vi "CODMn线性公式.vi"(0 "标液浓度":dbl[](array[numeric]), 1 "信号值":dbl[](array[numeric]), 4 "启用":bool[](array[boolean]), 5 "method":T1 caption="方法" items=["最小二乘", "最小绝对残差", "Bisquare"], 6 "模型":enum32{"线性", "多项式", "折线"}(ring), 7 "精度":i32=6) -> (13 "Polynomial Coefficients 2":dbl[](array[numeric]) caption="多项式系数2", 14 "拟合方程":string, 15 "r^2":dbl format="%.7g", 16 "拟合方程 2":string, 17 "r^2 2":dbl caption="r^2" format="%.7g", 18 "XY图":cluster{"X Values":dbl[], "Y Values":dbl[]}[](graph), 19 "Polynomial Coefficients":dbl[](array[numeric]) caption="多项式系数")   [LabVIEW 2016, in "斯坦道CODMn新电路板.lvlib"]
uses:
  <vilib>/Analysis/6fits.llb/Curve Fitting Criteria.ctl
  <vilib>/Analysis/NI_AALPro.lvlib
  <vilib>/gmath/NI_Gmath.lvlib
panel:
  out "Best Linear Fit 2":dbl[](array[numeric]) caption="最佳线性拟合2"
  out "Best Linear Fit":dbl[](array[numeric]) caption="最佳线性拟合"
  out "二维数组":dbl[][](array[numeric])
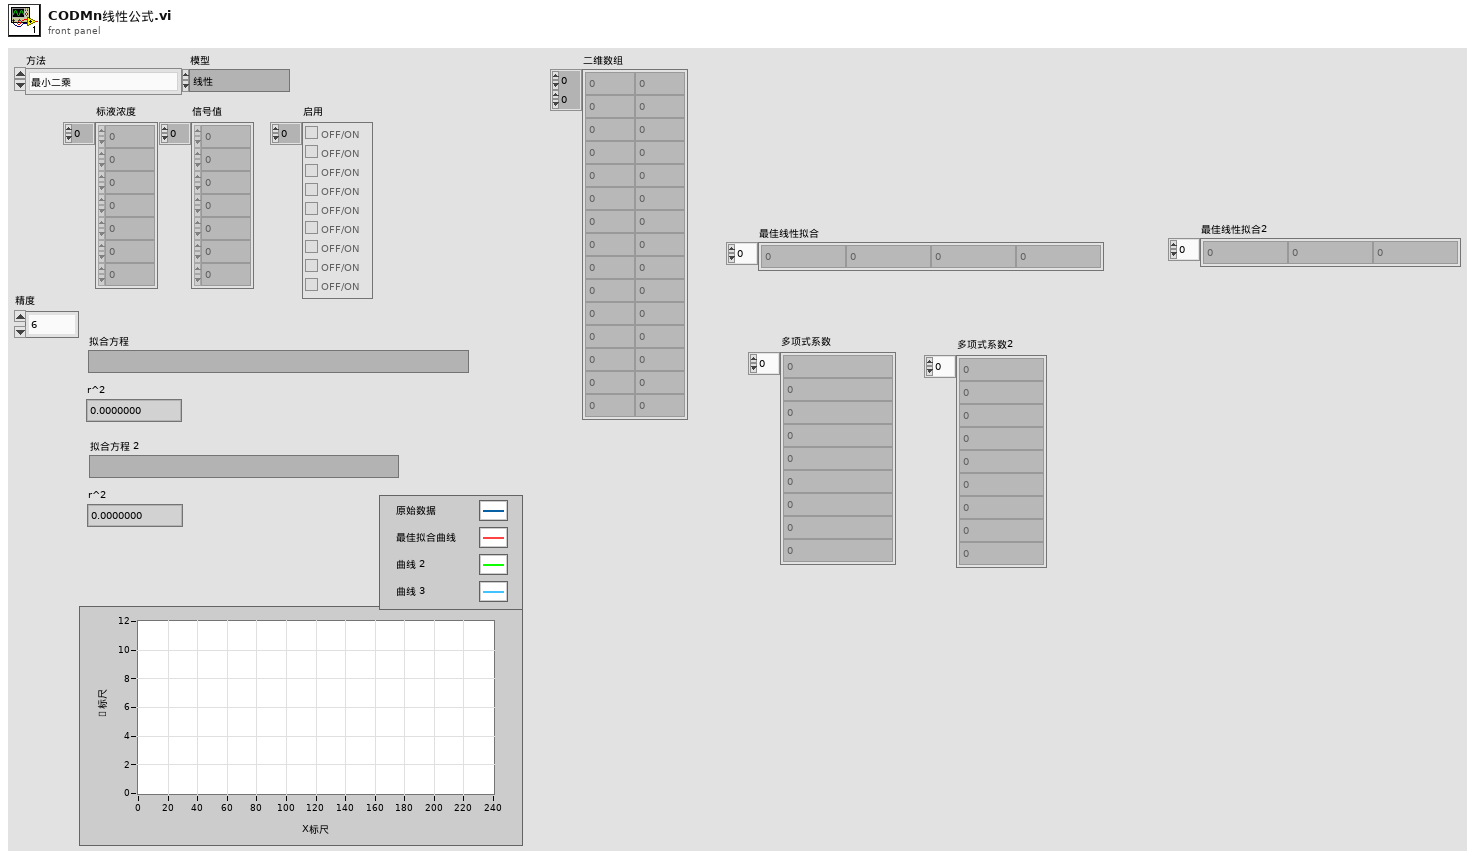
[diagram p1: front panel]
types:
  T1 = typedef "NI_AALPro.lvlib/Curve Fitting Criteria.ctl" = u16
  T2 = enum16{"Linear", "Polynomial", "Exponential", "Power"}
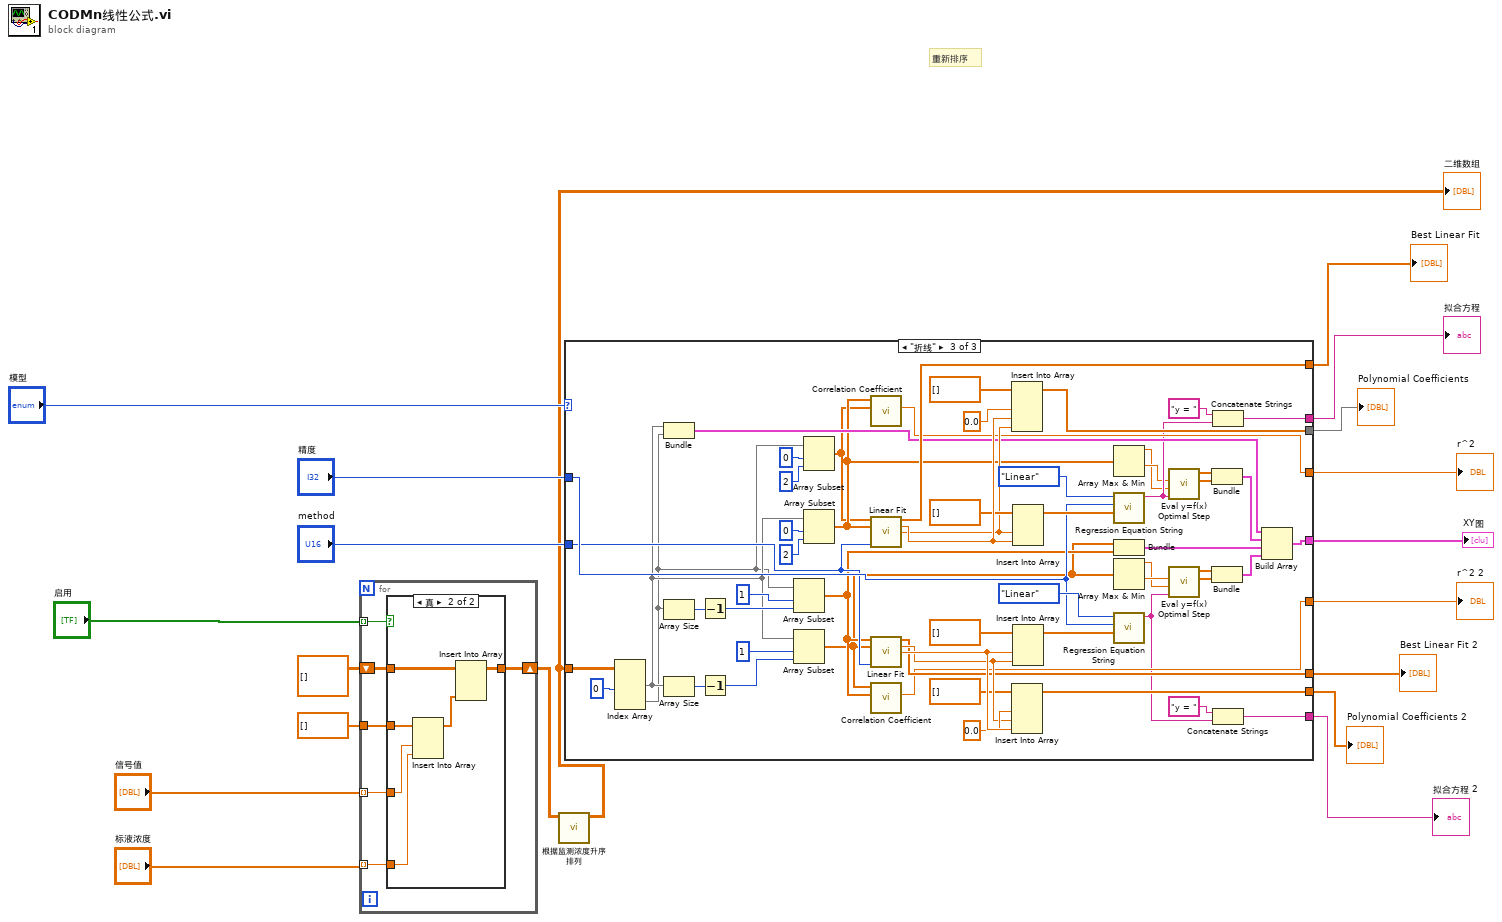
[diagram p0: block diagram]
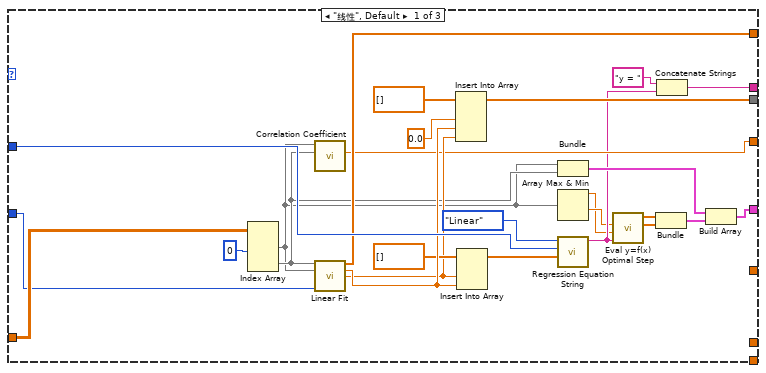
[diagram p2: hidden frame]
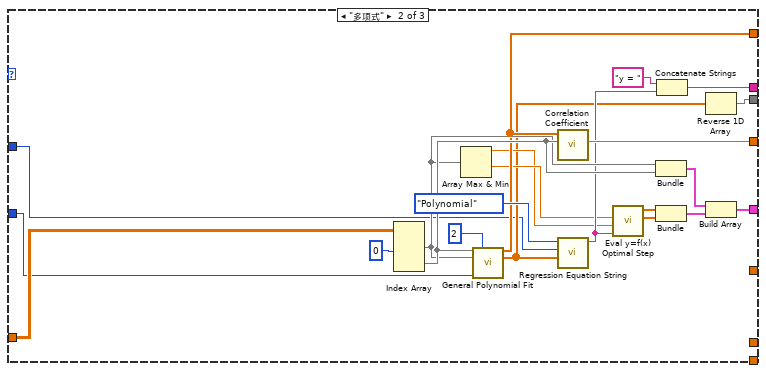
[diagram p3: hidden frame]
diagram:
  # "重新排序"
  n1 = for {
    tunnel: "启用" -> [w20] mode=indexing
    tunnel: "信号值" -> [w23] mode=indexing
    tunnel: "标液浓度" -> [w22] mode=indexing
    shift-right: [w21] -> w4
    shift-left: dbl[][] [] ("标液浓度") -> [w25]
    tunnel: dbl[] [] ("监测浓度") -> [w24]
    n2 = case shown="真" w20 {
      tunnel: w25 -> [w26 w32]
      tunnel: w24 -> [_ w31]
      tunnel: w23 -> [_ w30]
      tunnel: w22 -> [_ w29]
      tunnel: [w26 w27] -> w21
      frame False {
      }
      frame True {
        n3 = Insert Into Array(array=w31, new element #1=w30, new element #2=w29) -> (w28:dbl[])  [unwired: 1 in]
        n4 = Insert Into Array(array=w32, new element=w28) -> (w27:dbl[][])  [unwired: 2 in]
      }
    }
  }
  n5 = call "根据监测浓度升序排列.vi"("标液浓度输入"=w4) -> ("输出数组"=w3:dbl[][])  [unwired: 10 in]
  "二维数组" <- w3
  n6 = case shown="\"折线\"" "模型" {
    tunnel: w3 -> [w57 w73 w128]
    tunnel: "精度" -> [w50 w59 w106]
    tunnel: [w44 w64 w125] -> w15
    tunnel: [w43 w68 w124] -> w14
    tunnel: [w42 w71 w126] -> w13
    tunnel: [w41 w72 w127] -> w12
    tunnel: [w39 w69 w123] -> w11
    tunnel: "method" -> [w36 w65 w105]
    tunnel: [_ _ w110] -> w9
    tunnel: [_ _ w109] -> w8
    tunnel: [_ _ w108] -> w7
    tunnel: [_ _ w107] -> w6
    frame "线性", Default {
      n7 = Index Array(array=w57, index (col) #1=0 ("禁用的索引 (列)")) -> (element #1=w37:dbl[], element #2=w38:dbl[])  [unwired: 3 in]
      n8 = call <vilib>:"Correlation Coefficient.vi"("Y"=w38, "X"=w37) -> ("r^2"=w43:dbl)  [unwired: 8 in, 1 out]
      n9 = call <vilib>:"Linear Fit.vi"("Y"=w38, "X"=w37, "method"=w36) -> ("Best Linear Fit"=w44:dbl[], "slope"=w48:dbl, "intercept"=w45:dbl)  [unwired: 8 in, 2 out]
      n10 = Insert Into Array(array=dbl[] [] ("数组"), new element #1=0.0 ("新元素/子数组"), new element #2=w48, new element #3=w45) -> (w39:dbl[])  [unwired: 1 in]
      n11 = Insert Into Array(array=dbl[] [] ("数组"), new element #1=w45, new element #2=w48) -> (w40:dbl[])  [unwired: 1 in]
      n12 = Bundle("输出数组"=w37, "输出数组"=w38) -> (w54:cluster{"输出数组":dbl[], "输出数组":dbl[]})  [unwired: 1 in]
      n13 = Array Max & Min(array=w37) -> (max value=w33:dbl, min value=w34:dbl)  [unwired: 2 out]
      n14 = call "Regression Equation String.vi"("系数"=w40, "精度"=w50, "拟合类型"=T2."Linear") -> ("公式"=w35:string)  [unwired: 8 in]
      n15 = call <vilib>:"Eval y=f(x) Optimal Step.vi"("formula"=w35, "end"=w33, "start"=w34) -> ("Y Values"=w56:dbl[], "X Values"=w55:dbl[])  [unwired: 2 in, 2 out]
      n16 = Bundle("X Values"=w55, "Y Values"=w56) -> (w53:cluster{"X Values":dbl[], "Y Values":dbl[]})  [unwired: 1 in]
      n17 = Concatenate Strings("y = " ("string"), w35) -> (w42:string)
      n18 = Build Array(w54, w53) -> (w41:cluster{"X Values":dbl[], "Y Values":dbl[]}[])
    }
    frame "多项式" {
      n19 = Index Array(array=w73, index (col) #1=0 ("禁用的索引 (列)")) -> (element #1=w66:dbl[], element #2=w67:dbl[])  [unwired: 3 in]
      n20 = Array Max & Min(array=w66) -> (max value=w61:dbl, min value=w62:dbl)  [unwired: 2 out]
      n21 = call <vilib>:"General Polynomial Fit.vi"("Y"=w67, "polynomial order"=2, "X"=w66, "method"=w65) -> ("Best Polynomial Fit"=w64:dbl[], "Polynomial Coefficients"=w60:dbl[])  [unwired: 8 in, 2 out]
      n22 = call <vilib>:"Correlation Coefficient.vi"("Y"=w67, "X"=w64) -> ("r^2"=w68:dbl)  [unwired: 8 in, 1 out]
      n23 = call "Regression Equation String.vi"("系数"=w60, "精度"=w59, "拟合类型"=T2."Polynomial") -> ("公式"=w63:string)  [unwired: 8 in]
      n24 = call <vilib>:"Eval y=f(x) Optimal Step.vi"("formula"=w63, "end"=w61, "start"=w62) -> ("Y Values"=w79:dbl[], "X Values"=w78:dbl[])  [unwired: 2 in, 2 out]
      n25 = Bundle("输出数组"=w66, "输出数组"=w67) -> (w77:cluster{"输出数组":dbl[], "输出数组":dbl[]})  [unwired: 1 in]
      n26 = Bundle("X Values"=w78, "Y Values"=w79) -> (w76:cluster{"X Values":dbl[], "Y Values":dbl[]})  [unwired: 1 in]
      n27 = Concatenate Strings("y = " ("string"), w63) -> (w71:string)
      n28 = Reverse 1D Array(array=w60) -> (reversed array=w69:dbl[])
      n29 = Build Array(w77, w76) -> (w72:cluster{"X Values":dbl[], "Y Values":dbl[]}[])
    }
    frame "折线" {
      n30 = Index Array(array=w128, index (col) #1=0 ("禁用的索引 (列)")) -> (element #1=w82:dbl[], element #2=w81:dbl[])  [unwired: 3 in]
      n31 = Bundle("输出数组"=w82, "输出数组"=w81) -> (w98:cluster{"输出数组":dbl[], "输出数组":dbl[]})  [unwired: 1 in]
      n32 = Array Size(array=w81) -> (size(s)=w103:i32)
      n33 = Array Size(array=w82) -> (size(s)=w101:i32)
      n34 = Decrement(x=w103) -> (x-1=w102:i32)
      n35 = Decrement(x=w101) -> (x-1=w99:i32)
      n36 = Array Subset(array=w81, index=1 ("索引"), length=w102) -> (w97:dbl[])
      n37 = Array Subset(array=w82, index=1 ("索引"), length=w99) -> (w90:dbl[])
      n38 = Array Subset(array=w81, index=0 ("索引"), length=2 ("长度")) -> (w87:dbl[])
      n39 = Array Subset(array=w82, index=0 ("索引"), length=2 ("长度")) -> (w88:dbl[])
      n40 = call <vilib>:"Correlation Coefficient.vi"("Y"=w87, "X"=w88) -> ("r^2"=w124:dbl)  [unwired: 8 in, 1 out]
      n41 = call <vilib>:"Linear Fit.vi"("Y"=w87, "X"=w88, "method"=w105) -> ("Best Linear Fit"=w125:dbl[], "slope"=w133:dbl, "intercept"=w130:dbl)  [unwired: 8 in, 2 out]
      n42 = call <vilib>:"Linear Fit.vi"("Y"=w97, "X"=w90, "method"=w105) -> ("Best Linear Fit"=w110:dbl[], "slope"=w114:dbl, "intercept"=w117:dbl)  [unwired: 8 in, 2 out]
      n43 = call <vilib>:"Correlation Coefficient.vi"("Y"=w97, "X"=w90) -> ("r^2"=w109:dbl)  [unwired: 8 in, 1 out]
      n44 = Insert Into Array(array=dbl[] [] ("数组"), new element #1=0.0 ("新元素/子数组"), new element #2=w133, new element #3=w130) -> (w123:dbl[])  [unwired: 1 in]
      n45 = Insert Into Array(array=dbl[] [] ("数组"), new element #1=0.0 ("新元素/子数组"), new element #2=w114, new element #3=w117) -> (w107:dbl[])  [unwired: 1 in]
      n46 = Insert Into Array(array=dbl[] [] ("数组"), new element #1=w130, new element #2=w133) -> (w129:dbl[])  [unwired: 1 in]
      n47 = Insert Into Array(array=dbl[] [] ("数组"), new element #1=w117, new element #2=w114) -> (w118:dbl[])  [unwired: 1 in]
      n48 = Array Max & Min(array=w88) -> (max value=w85:dbl, min value=w86:dbl)  [unwired: 2 out]
      n49 = call "Regression Equation String.vi"("系数"=w129, "精度"=w106, "拟合类型"=T2."Linear") -> ("公式"=w96:string)  [unwired: 8 in]
      n50 = Bundle(w90, w97) -> (w91:cluster{dbl[], dbl[]})  [unwired: 1 in]
      n51 = Array Max & Min(array=w90) -> (max value=w83:dbl, min value=w84:dbl)  [unwired: 2 out]
      n52 = call "Regression Equation String.vi"("系数"=w118, "精度"=w106, "拟合类型"=T2."Linear") -> ("公式"=w89:string)  [unwired: 8 in]
      n53 = call <vilib>:"Eval y=f(x) Optimal Step.vi"("formula"=w96, "end"=w85, "start"=w86) -> ("Y Values"=w138:dbl[], "X Values"=w137:dbl[])  [unwired: 2 in, 2 out]
      n54 = call <vilib>:"Eval y=f(x) Optimal Step.vi"("formula"=w89, "end"=w83, "start"=w84) -> ("Y Values"=w94:dbl[], "X Values"=w95:dbl[])  [unwired: 2 in, 2 out]
      n55 = Bundle("X Values"=w137, "Y Values"=w138) -> (w92:cluster{"X Values":dbl[], "Y Values":dbl[]})  [unwired: 1 in]
      n56 = Bundle("X Values"=w95, "Y Values"=w94) -> (w93:cluster{"X Values":dbl[], "Y Values":dbl[]})  [unwired: 1 in]
      n57 = Concatenate Strings("y = " ("string"), w96) -> (w126:string)
      n58 = Concatenate Strings("y = " ("string"), w89) -> (w108:string)
      n59 = Build Array(w98, w92, w91, w93) -> (w127:cluster{"X Values":dbl[], "Y Values":dbl[]}[])
    }
  }
  "Best Linear Fit" <- w15
  "r^2" <- w14
  "拟合方程" <- w13
  "XY图" <- w12
  "Polynomial Coefficients" <- w11
  "r^2 2" <- w8
  "拟合方程 2" <- w7
  "Best Linear Fit 2" <- w9
  "Polynomial Coefficients 2" <- w6
